vi "Start Log.vi"(8 "error in (no error)":errorcluster, 9 "Timestamp data points":bool, 10 "tdms file":refnum<k34>, 11 "Acquired Result in":refnum<class "Acquired Result.lvclass">) -> (0 "error out":errorcluster, 2 "tdms file out":refnum<k34>, 3 "Acquired Result out":refnum<class "Acquired Result.lvclass">)   [LabVIEW 2018, in "Acquired Result.lvclass"]
uses:
  Acquired Result.lvclass
  Acquired Result.lvclass/Acquired Result.ctl
  Read Group.vi
  Read Channels.vi
  Read Settings.vi
  Read Time group.vi
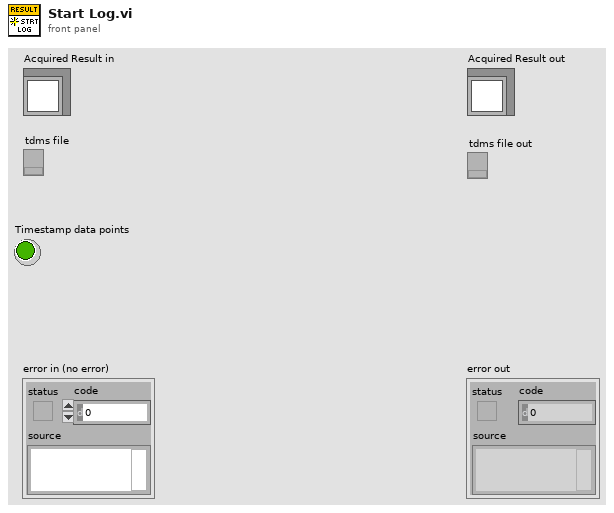
[diagram p1: front panel]
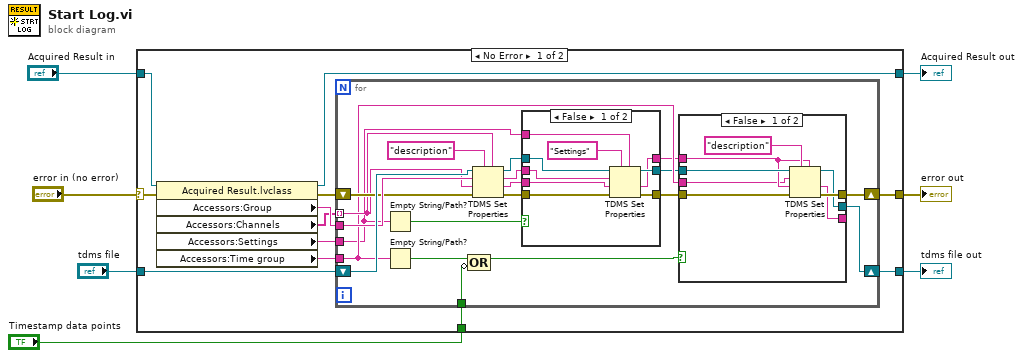
[diagram p0: block diagram]
diagram:
  n1 = case shown="No Error" "error in (no error)" {
    selector: "error in (no error)" -> [w12 w65]
    tunnel: [w18 w65] -> w6
    tunnel: [w13 w64] -> w4
    tunnel: "Acquired Result in" -> [w14 w64]
    tunnel: "tdms file" -> [w16 w63]
    tunnel: [w15 w63] -> w2
    tunnel: "Timestamp data points" -> [w8 _]
    frame No Error {
      n2 = property class="Acquired Result.lvclass"(reference=w14, error in=w12) -> (reference out=w13:refnum<class "Acquired Result.lvclass">, error out=w11:errorcluster, "Accessors:Group"=w19:string, "Accessors:Channels"=w17:string[], "Accessors:Settings"=w10:string, "Accessors:Time group"=w9:string)
      n3 = for {
        tunnel: w19 -> [w38]
        shift-right: [w23] -> w15
        shift-left: w16 -> [w39]
        shift-right: [w24] -> w18
        shift-left: w11 -> [w37]
        tunnel: w17 -> [w34] mode=indexing
        tunnel: w10 -> [w22]
        tunnel: w9 -> [w33]
        tunnel: w8 -> [w20]
        n4 = Empty String/Path?(string/path=w22) -> (empty?=w27:bool)
        n5 = Empty String/Path?(string/path=w33) -> (empty?=w35:bool)
        n6 = Compound Arithmetic op=OR(w35, invert w20) -> (w21:bool)
        n7 = TDMS Set Properties(5:w34, 7:"description", 8:w37, 9:w34, 10:w38, 11:w39) -> (0:w29:errorcluster, 1:w30:string, 2:w32:string, 3:w31:refnum<k34>)
        n8 = case shown="False" w27 {
          tunnel: w31 -> [w48 w51]
          tunnel: w29 -> [w47 w50]
          tunnel: [w46 w50] -> w25
          tunnel: [w45 w51] -> w26
          tunnel: w30 -> [w43 w49]
          tunnel: w32 -> [w42 _]
          tunnel: [w41 w49] -> w28
          tunnel: w22 -> [w40 _]
          frame False {
            n9 = TDMS Set Properties(5:w40, 7:"Settings", 8:w47, 9:w43, 10:w42, 11:w48) -> (0:w46:errorcluster, 1:w41:string, 3:w45:refnum<k34>)  [unwired: 1 out]
          }
          frame True {
          }
        }
        n10 = case shown="False" w21 {
          tunnel: w26 -> [w59 w62]
          tunnel: w25 -> [w58 w61]
          tunnel: [w57 w61] -> w24
          tunnel: [w56 w62] -> w23
          tunnel: w28 -> [w54 w60]
          tunnel: w33 -> [w53 _]
          tunnel: [w52 w60] -> _
          frame False {
            n11 = TDMS Set Properties(5:w54, 7:"description", 8:w58, 9:w54, 10:w53, 11:w59) -> (0:w57:errorcluster, 1:w52:string, 3:w56:refnum<k34>)  [unwired: 1 out]
          }
          frame True {
          }
        }
      }
    }
    frame Error {
    }
  }
  "error out" <- w6
  "Acquired Result out" <- w4
  "tdms file out" <- w2
